vi "Days of Month.vi"(8 "error in (no error)":errorcluster, 10 "YYYY : Year string, empty will use current year":string, 11 "Month":i32=1 min=1 max=12 step=1) -> (0 "error out":errorcluster, 3 "Days of Month":i32[](array[numeric]))   [LabVIEW 2021]
doc: "get the days array of month.\n\nif YYYY input year is empty will use current year"
uses:
  <userlib>/_OpenG.lib/array/array.llb/Search 1D Array (I32)__ogtk.vi
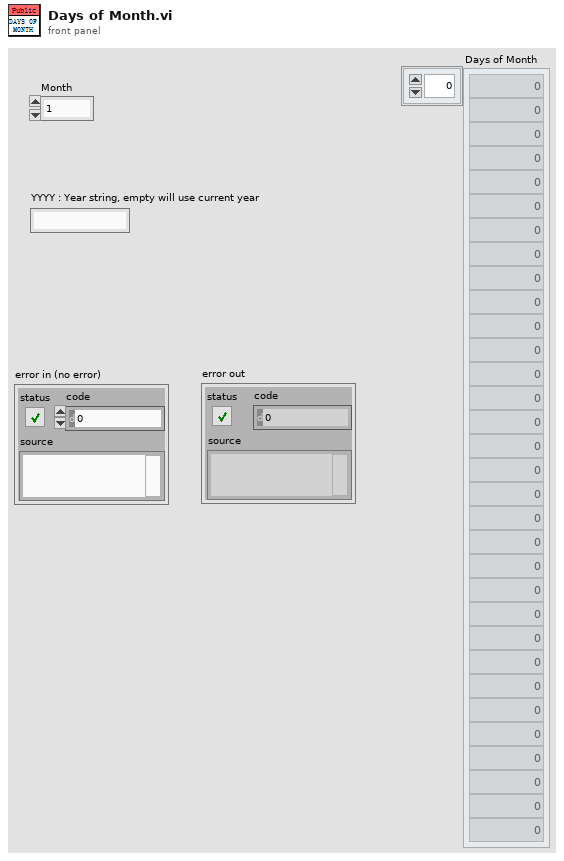
[diagram p1: front panel]
types:
  T1 = typedef "LVDateTimeRec.ctl" = cluster{"fractional second":dbl, "second":i32, "minute":i32, "hour":i32, "day of month":i32, "month":i32, "year":i32, "day of week":i32, "day of year":i32, "DST":i32}
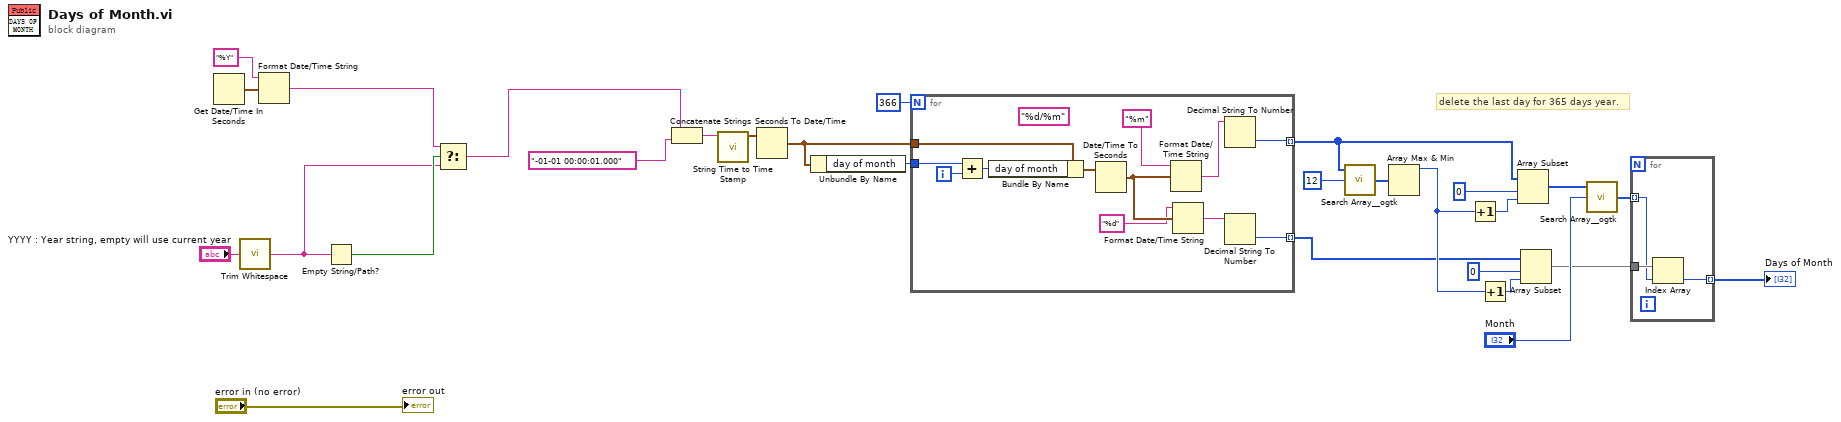
[diagram p0: block diagram]
diagram:
  # "delete the last day for 365 days year."
  n1 = Get Date/Time In Seconds() -> (seconds since 1Jan1904=w15:timestamp)
  n2 = call <vilib>:"Trim Whitespace.vi"("string"="YYYY : Year string, empty will use current year") -> ("trimmed string"=w1:string)  [unwired: 1 in]
  n3 = Format Date/Time String(time format string (%c)="%Y", seconds (now)=w15) -> (date/time string=w3:string)  [unwired: 1 in]
  n4 = Empty String/Path?(string/path=w1) -> (empty?=w4:bool)
  n5 = Select(t=w3, s=w4, f=w1) -> (s? t:f=w2:string)
  n6 = Concatenate Strings(w2, "-01-01 00:00:01.000" ("string")) -> (w13:string)
  n7 = call "String Time to Time Stamp.vi"("input TimeStamp string"=w13) -> ("Time Stamp"=w11:timestamp)  [unwired: 9 in, 1 out]
  n8 = Seconds To Date/Time(time stamp (now)=w11) -> (date time rec=w18:T1)  [unwired: 1 in]
  n9 = Unbundle By Name(w18) -> ("day of month"=w17:i32)
  n10 = for {
    N: 366 -> [_]
    tunnel: w18 -> [w40]
    tunnel: w17 -> [w39]
    tunnel: [w31] -> w22 mode=indexing
    tunnel: [w29] -> w27 mode=indexing
    i -> [w38]
    (unwired) "%d/%m" ("time format string (%c)")
    n11 = Add(x=w39, y=w38) -> (x+y=w37:i32)
    n12 = Bundle By Name(cluster=w40, "day of month"=w37) -> (w36:T1)
    n13 = Date/Time To Seconds(2:w36) -> (0:w34:timestamp)  [unwired: 1 in]
    n14 = Format Date/Time String(time format string (%c)="%m", seconds (now)=w34) -> (date/time string=w32:string)  [unwired: 1 in]
    n15 = Format Date/Time String(time format string (%c)="%d", seconds (now)=w34) -> (date/time string=w30:string)  [unwired: 1 in]
    n16 = Decimal String To Number(string=w32) -> (number=w31:i32)  [unwired: 2 in, 1 out]
    n17 = Decimal String To Number(string=w30) -> (number=w29:i32)  [unwired: 2 in, 1 out]
  }
  n18 = call-poly <userlib>:"Search Array__ogtk.vi"("Array"=w22, "Element Data"=12) -> ("Indices of Elements"=w21:i32[])  [unwired: 7 in]
  n19 = Array Max & Min(array=w21) -> (max value=w28:i32)  [unwired: 3 out]
  n20 = Increment(x=w28) -> (x+1=w24:i32)
  n21 = Increment(x=w28) -> (x+1=w25:i32)
  n22 = Array Subset(array=w22, index=0, length=w24) -> (w10:i32[])
  n23 = Array Subset(array=w27, index=0, length=w25) -> (w7:i32[])
  n24 = call-poly <userlib>:"Search Array__ogtk.vi"("Array"=w10, "Element Data"="Month") -> ("Indices of Elements"=w8:i32[])  [unwired: 7 in]
  n25 = for {
    tunnel: w8 -> [w42] mode=indexing
    tunnel: w7 -> [w43]
    tunnel: [w41] -> w6 mode=indexing
    n26 = Index Array(array=w43, index=w42) -> (element=w41:i32)
  }
  "Days of Month" <- w6
  "error out" <- "error in (no error)"
